vi "Zapisz TDMS FVG.vi"(6 "Aktywacja":bool, 7 "Akcja":T4, 8 "error in (no error)":errorcluster, 9 "Group Data":T2, 10 "Przebiegi in":T1, 11 "File Data":T3) -> (0 "error out":errorcluster, 2 "Przebiegi out":T1)   [LabVIEW 2014]
doc: "Tworzy i zarządza plikiem danych TDMS"
uses:
  Kontrolki/FVGs/TDMS FVG.ctl
  Kontrolki/FVGs/TDMS File dane FVG.ctl
  Kontrolki/FVGs/TDMS Group dane FVG.ctl
  Kontrolki/Przetwarzanie/Kanaly.ctl
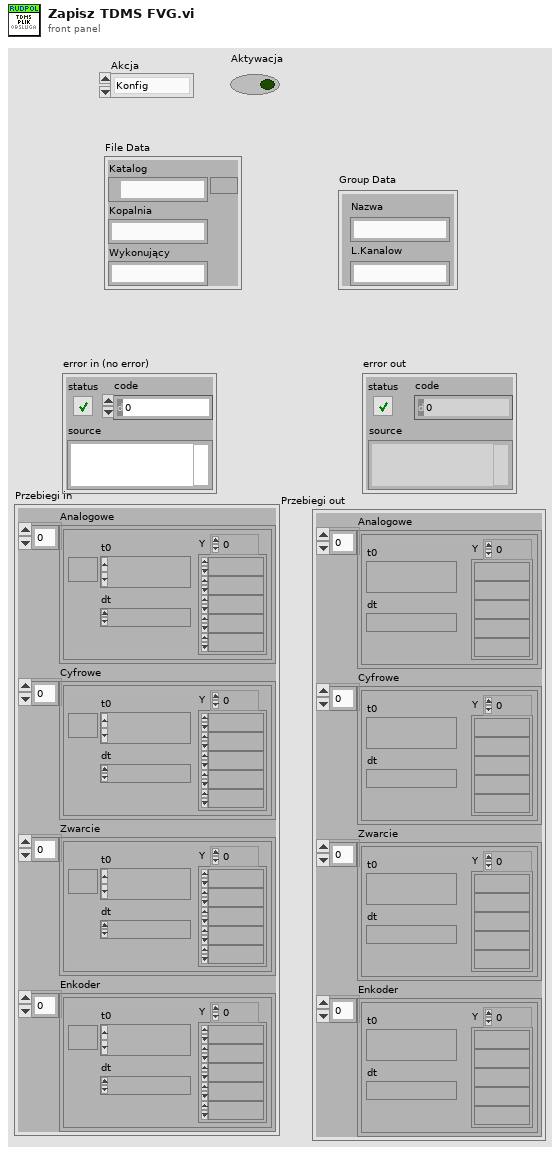
[diagram p1: front panel]
types:
  T1 = typedef "Kanaly.ctl" = cluster{"Analogowe":waveform(dbl)[], "Cyfrowe":waveform(dbl)[], "Zwarcie":waveform(dbl)[], "Enkoder":waveform(dbl)[]}
  T2 = typedef "TDMS Group dane FVG.ctl" = cluster{"Nazwa":string, "L.Kanalow":string}
  T3 = typedef "TDMS File dane FVG.ctl" = cluster{"Katalog":path, "Kopalnia":string, "Wykonujący":string}
  T4 = typedef "TDMS FVG.ctl" = enum16{"Konfig", "Dodaj Grupe", "Koniec"}
  T5 = enum16{"open", "open or create", "create or replace", "create", "open (read-only)"}
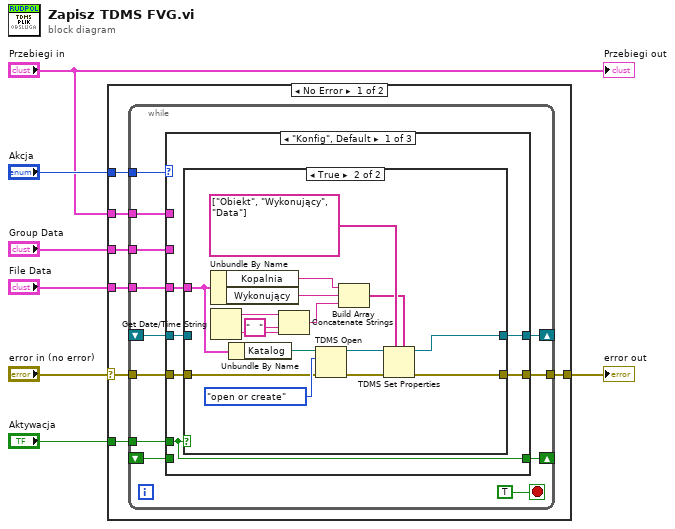
[diagram p0: block diagram]
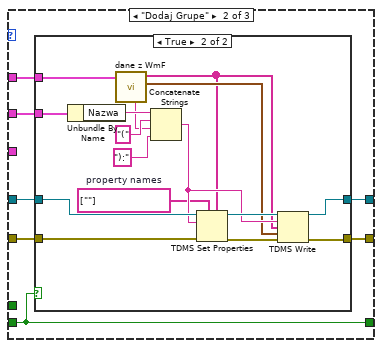
[diagram p3: hidden frame]
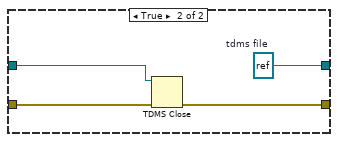
[diagram p6: hidden frame]
diagram:
  n1 = case shown="No Error" "error in (no error)" {
    selector: "error in (no error)" -> [w11 w87]
    tunnel: [w10 w87] -> w6
    tunnel: "Akcja" -> [w14 _]
    tunnel: "Aktywacja" -> [w13 _]
    tunnel: "File Data" -> [w12 _]
    tunnel: "Group Data" -> [w9 _]
    tunnel: "Przebiegi in" -> [w8 _]
    frame No Error {
      n2 = while {
        tunnel: w14 -> [w25]
        tunnel: w13 -> [w24]
        shift-right: [w23] -> _
        shift-left: _ -> [w22]
        tunnel: w12 -> [w21]
        tunnel: w11 -> [w20]
        tunnel: [w19] -> w10
        shift-right: [w18] -> _
        shift-left: _ -> [w17]
        tunnel: w9 -> [w16]
        tunnel: w8 -> [w15]
        stop <- TRUE stop-if-true
        n3 = case shown="\"Konfig\", Default" w25 {
          tunnel: w24 -> [w32 _ _]
          tunnel: [w32 w57 w80] -> w23
          tunnel: w22 -> [_ w57 w80]
          tunnel: w21 -> [w31 _ _]
          tunnel: w20 -> [w30 w56 w79]
          tunnel: [w29 w55 w77] -> w19
          tunnel: [w28 w54 w76] -> w18
          tunnel: w17 -> [w27 w53 w78]
          tunnel: w16 -> [_ w52 _]
          tunnel: w15 -> [_ w51 _]
          frame "Konfig", Default {
            n4 = case shown="True" w32 {
              tunnel: w31 -> [_ w36]
              tunnel: w30 -> [w34 w49]
              tunnel: [w34 w47] -> w29
              tunnel: [w33 w45] -> w28
              tunnel: w27 -> [w33 _]
              frame False {
              }
              frame True {
                n5 = Unbundle By Name(w36) -> ("Kopalnia"=w40:string, "Wykonujący"=w39:string)
                n6 = Get Date/Time String() -> (date string=w43:string, time string=w42:string)  [unwired: 3 in]
                n7 = Unbundle By Name(w36) -> ("Katalog"=w35:path)
                n8 = Concatenate Strings(w43, "   " ("string"), w42) -> (w38:string)
                n9 = TDMS Open(8:w49, 10:T5."open or create" ("operation (0:open)"), 11:w35) -> (0:w48:errorcluster, 3:w46:refnum<k34>)  [unwired: 4 in]
                n10 = Build Array(w40, w39, w38) -> (w37:string[])
                n11 = TDMS Set Properties(5:w37, 7:string[] ["Obiekt", "Wykonujący", "Data"], 8:w48, 11:w46) -> (0:w47:errorcluster, 3:w45:refnum<k34>)  [unwired: 2 in, 2 out]
              }
            }
          }
          frame "Dodaj Grupe" {
            n12 = case shown="True" w57 {
              tunnel: w56 -> [w59 w75]
              tunnel: [w59 w68] -> w55
              tunnel: [w58 w66] -> w54
              tunnel: w53 -> [w58 w74]
              tunnel: w52 -> [_ w73]
              tunnel: w51 -> [_ w64]
              frame False {
              }
              frame True {
                w62 = string[] [""]  # property names
                n13 = Unbundle By Name(w73) -> ("Nazwa"=w72:string)
                n14 = call "dane z WmF.vi"("Przebiegi in"=w64) -> ("przebiegi"=w63:waveform(dbl)[], "Nazwy"=w60:string[], "Kanaly"=w61:string)  [unwired: 6 in, 2 out]
                n15 = Concatenate Strings(w72, "(" ("string"), w61, "):" ("string")) -> (w65:string)
                n16 = TDMS Set Properties(5:w60, 7:w62, 8:w75, 10:w65, 11:w74) -> (0:w69:errorcluster, 3:w67:refnum<k34>)  [unwired: 1 in, 2 out]
                n17 = TDMS Write(0:w67, 5:w65, 7:w60, 9:w63, 11:w69) -> (4:w66:refnum<k34>, 15:w68:errorcluster)  [unwired: 1 in, 2 out]
              }
            }
          }
          frame "Koniec" {
            n18 = case shown="False" w80 {
              tunnel: w79 -> [w82 w86]
              tunnel: w78 -> [w81 w83]
              tunnel: [w82 w85] -> w77
              tunnel: [w81 w84] -> w76
              frame False {
              }
              frame True {
                w84 = refnum<k34> refnum  # tdms file
                n19 = TDMS Close(8:w86, 11:w83) -> (0:w85:errorcluster)  [unwired: 1 out]
              }
            }
          }
        }
      }
    }
    frame Error {
    }
  }
  "error out" <- w6
  "Przebiegi out" <- "Przebiegi in"
